vi "data_subset.vi"(8 "error in (no error)":errorcluster, 9 "length":u64, 10 "index":u64, 11 "data":T1) -> (0 "error out":errorcluster, 3 "data subset":T1)   [LabVIEW 2017, in "NI_ExcelFile.lvlib"]
uses:
  <vilib>/express/express shared/NI_ExcelFile/NI_ExcelFile.lvlib
  <vilib>/express/express shared/NI_ExcelFile/Ctrls/data_AllTypeData.ctl
  <vilib>/express/express shared/NI_ExcelFile/Ctrls/DataType.ctl
  <vilib>/express/express shared/NI_ExcelFile/SubVIs/utilities_addTime.vi
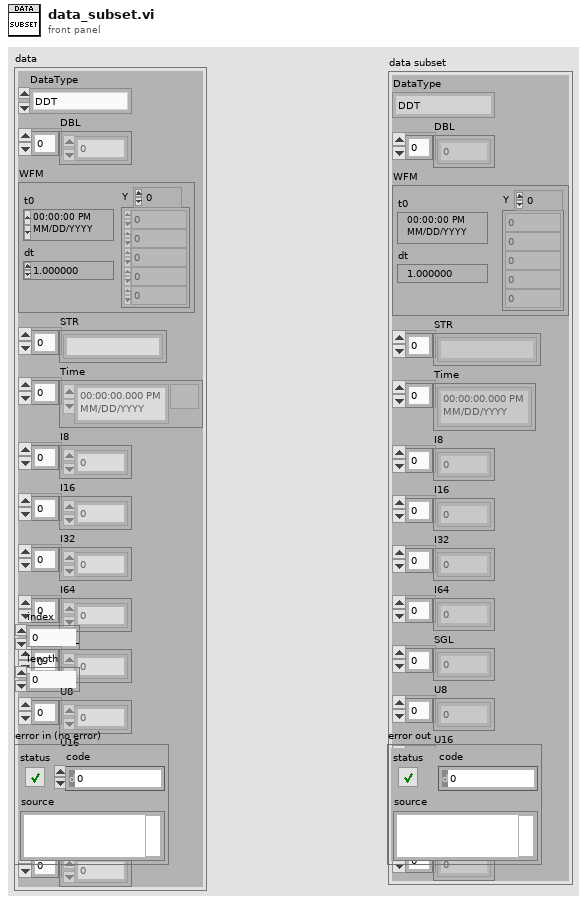
[diagram p1: front panel]
types:
  T1 = typedef "NI_ExcelFile.lvlib/data_AllTypeData.ctl" = cluster{"DataType":T2, "DBL":dbl[], "WFM":waveform(dbl), "STR":string[], "Time":timestamp[], "I8":i8[], "I16":i16[], "I32":i32[], "I64":i64[], "SGL":sgl[], "U8":u8[], "U16":u16[], "U32":u32[], "U64":u64[]}
  T2 = typedef "NI_ExcelFile.lvlib/DataType.ctl" = enum16{"DDT", "WFM", "Array of STR", "Array of DBL", "Array of I8", "Array of I16", "Array of I32", "Array of I64", "Array of SGL", "Array of U8", "Array of U16", "Array of U32", "Array of U64", "Array of Time"}
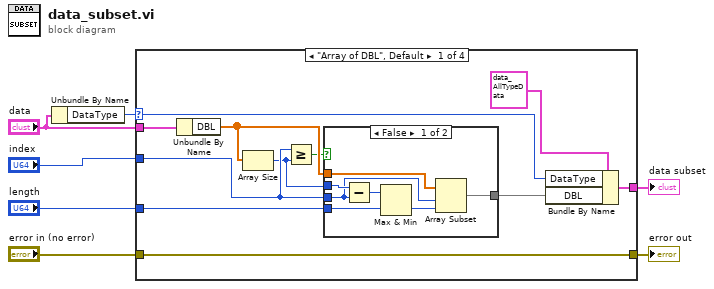
[diagram p0: block diagram]
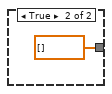
[diagram p2: hidden frame]
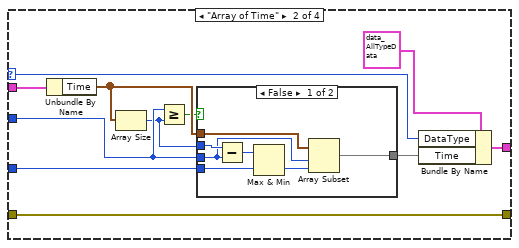
[diagram p3: hidden frame]
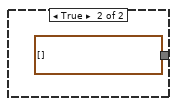
[diagram p4: hidden frame]
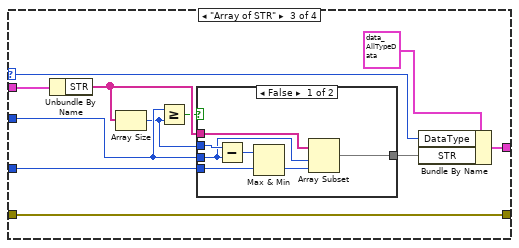
[diagram p5: hidden frame]
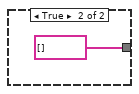
[diagram p6: hidden frame]
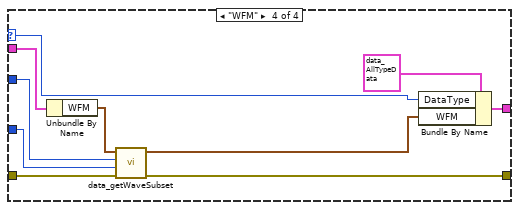
[diagram p7: hidden frame]
diagram:
  n1 = Unbundle By Name("data") -> ("DataType"=w7:T2)
  n2 = case shown="\"Array of DBL\", Default" w7 {
    selector: w7 -> [w14 w33 w52 w72]
    tunnel: "data" -> [w18 w37 w56 w74]
    tunnel: "index" -> [w11 w30 w49 w69]
    tunnel: "length" -> [w17 w36 w55 w68]
    tunnel: [w16 w35 w54 w71] -> w2
    tunnel: "error in (no error)" -> [w13 w32 w51 w67]
    tunnel: [w13 w32 w51 w66] -> w1
    frame "Array of DBL", Default {
      n3 = Unbundle By Name(w18) -> ("DBL"=w12:dbl[])
      n4 = Array Size(array=w12) -> (size(s)=w10:i32)
      n5 = Greater Or Equal?(x=w11, y=w10) -> (x >= y?=w8:bool)
      n6 = case shown="False" w8 {
        tunnel: w17 -> [w22 _]
        tunnel: [w25 dbl[] []] -> w9
        tunnel: w12 -> [w19 _]
        tunnel: w11 -> [w20 _]
        tunnel: w10 -> [w24 _]
        frame False {
          n7 = Subtract(x=w24, y=w20) -> (x-y=w23:u64)
          n8 = Max & Min(x=w23, y=w22) -> (min(x,y)=w21:u64)  [unwired: 1 out]
          n9 = Array Subset(array=w19, index=w20, length=w21) -> (w25:dbl[])
        }
        frame True {
        }
      }
      n10 = Bundle By Name(cluster=T1 {"DataType"=enum."DDT", "DBL"=[], "WFM"={"t0"=timestamp(0 s since 1904-01-01), "dt"=1.0, "Y"=[]}, "STR"=[], "Time"=[], "I8"=[], "I16"=[], "I32"=[], "I64"=[], "SGL"=[], "U8"=[], "U16"=[], "U32"=[], "U64"=[]} ("data"), "DataType"=w14, "DBL"=w9) -> (w16:T1)
    }
    frame "Array of Time" {
      n11 = Unbundle By Name(w37) -> ("Time"=w31:timestamp[])
      n12 = Array Size(array=w31) -> (size(s)=w29:i32)
      n13 = Greater Or Equal?(x=w30, y=w29) -> (x >= y?=w27:bool)
      n14 = case shown="False" w27 {
        tunnel: w36 -> [w41 _]
        tunnel: [w44 timestamp[] []] -> w28
        tunnel: w31 -> [w38 _]
        tunnel: w30 -> [w39 _]
        tunnel: w29 -> [w43 _]
        frame False {
          n15 = Subtract(x=w43, y=w39) -> (x-y=w42:u64)
          n16 = Max & Min(x=w42, y=w41) -> (min(x,y)=w40:u64)  [unwired: 1 out]
          n17 = Array Subset(array=w38, index=w39, length=w40) -> (w44:timestamp[])
        }
        frame True {
        }
      }
      n18 = Bundle By Name(cluster=T1 {"DataType"=enum."DDT", "DBL"=[], "WFM"={"t0"=timestamp(0 s since 1904-01-01), "dt"=1.0, "Y"=[]}, "STR"=[], "Time"=[], "I8"=[], "I16"=[], "I32"=[], "I64"=[], "SGL"=[], "U8"=[], "U16"=[], "U32"=[], "U64"=[]} ("data"), "DataType"=w33, "Time"=w28) -> (w35:T1)
    }
    frame "Array of STR" {
      n19 = Unbundle By Name(w56) -> ("STR"=w50:string[])
      n20 = Array Size(array=w50) -> (size(s)=w48:i32)
      n21 = Greater Or Equal?(x=w49, y=w48) -> (x >= y?=w46:bool)
      n22 = case shown="False" w46 {
        tunnel: w55 -> [w60 _]
        tunnel: [w63 string[] []] -> w47
        tunnel: w50 -> [w57 _]
        tunnel: w49 -> [w58 _]
        tunnel: w48 -> [w62 _]
        frame False {
          n23 = Subtract(x=w62, y=w58) -> (x-y=w61:u64)
          n24 = Max & Min(x=w61, y=w60) -> (min(x,y)=w59:u64)  [unwired: 1 out]
          n25 = Array Subset(array=w57, index=w58, length=w59) -> (w63:string[])
        }
        frame True {
        }
      }
      n26 = Bundle By Name(cluster=T1 {"DataType"=enum."DDT", "DBL"=[], "WFM"={"t0"=timestamp(0 s since 1904-01-01), "dt"=1.0, "Y"=[]}, "STR"=[], "Time"=[], "I8"=[], "I16"=[], "I32"=[], "I64"=[], "SGL"=[], "U8"=[], "U16"=[], "U32"=[], "U64"=[]} ("data"), "DataType"=w52, "STR"=w47) -> (w54:T1)
    }
    frame "WFM" {
      n27 = Unbundle By Name(w74) -> ("WFM"=w70:waveform(dbl))
      n28 = call <vilib>:"data_getWaveSubset.vi"("error in (no error)"=w67, "length"=w68, "index"=w69, "Waveform"=w70) -> ("error out"=w66:errorcluster, "Waveform out"=w65:waveform(dbl))  [unwired: 6 in]
      n29 = Bundle By Name(cluster=T1 {"DataType"=enum."DDT", "DBL"=[], "WFM"={"t0"=timestamp(0 s since 1904-01-01), "dt"=1.0, "Y"=[]}, "STR"=[], "Time"=[], "I8"=[], "I16"=[], "I32"=[], "I64"=[], "SGL"=[], "U8"=[], "U16"=[], "U32"=[], "U64"=[]} ("data"), "DataType"=w72, "WFM"=w65) -> (w71:T1)
    }
  }
  "data subset" <- w2
  "error out" <- w1
